vi "LIA DFD Decimation.vi"(7 "stages":i32, 9 "filter delay":i32, 10 "filter in":T1 {"mSRate_QSettings"."source" items=["Coef a/k"=0, "Coef b/v"=7, "Input"=1, "Output"=2, "Multiplicand"=3, "Product"=4, "Sum"=5, "Delay"=6, "Gain"=8]}, 11 "data in":cdb[](array[numeric])) -> (2 "total decimation":dbl, 3 "decimated data":cdb[](array[numeric]))   [LabVIEW 2017]
uses:
  <vilib>/addons/Digital Filter Design/_Objects.llb/DFD Filter Obj.ctl
  <vilib>/addons/Digital Filter Design/_Objects.llb/DFD Filter Coef.ctl
  <vilib>/addons/Digital Filter Design/_Objects.llb/DFD Filter Structure Type Selector.ctl
  <vilib>/addons/Digital Filter Design/_Objects.llb/dfd_Internal Quantization Settings.ctl
  <vilib>/addons/Digital Filter Design/_Objects.llb/dfd_Internal Quantization Srcs.ctl
  <vilib>/addons/Digital Filter Design/_Objects.llb/DFD Coef Norm Type.ctl
  <vilib>/Analysis/2dsp.llb/Decimate (single shot, CDB).vi
  <vilib>/addons/Digital Filter Design/Process.llb/DFD Filtering (Array).vi
  <vilib>/addons/Digital Filter Design/NI_DigFilterLicensed.lvlib
  <vilib>/Analysis/NI_AALPro.lvlib
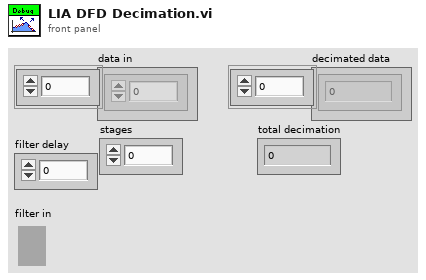
[diagram p1: front panel]
types:
  T1 = typedef "NI_DigFilterLicensed.lvlib/DFD Filter Obj.ctl" = cluster{"mSRate_Fs":dbl, "mSRate_Version":string, "mSRate_Comments":string, "mSRate_OrgCoef":T2, "mSRate_CurCoef":T2, "mSRate_Quantized?":bool, "mSRate_QCoef":T2, "mSRate_QSettings":T4[], "mSRate_Order":i32, "mSRate_Scaling":cluster{"mSRate_ScaleByPowerOf2?":bool, "mSRate_ScaleType":T6}}
  T2 = typedef "NI_DigFilterLicensed.lvlib/DFD Filter Coef.ctl" = cluster{"type":T3, "gain":dbl, "coef a (k)":dbl[], "coef b (v)":dbl[]}
  T3 = typedef "NI_DigFilterLicensed.lvlib/DFD Filter Structure Type Selector.ctl" = enum16{"Undefined", "FIR Direct Form", "FIR Direct Form Transposed", "FIR Symmetric", "FIR Antisymmetric", "IIR Direct Form I", "IIR Direct Form I Transposed", "IIR Direct Form II", "IIR Direct Form II Transposed", "IIR Cascaded Second Order Sections Form I", "IIR Cascaded Second Order Sections Form I Transposed", "IIR Cascaded Second Order Sections Form II", "IIR Cascaded Second Order Sections Form II Transposed", "Lattice Allpass (basic sections)", "Lattice Allpass (one multiplier sections)", "Lattice Allpass (normalized sections)", "Lattice AR (basic sections)", "Lattice AR (one multiplier sections)", "Lattice AR (normalized sections)", "Lattice MA (minimum phase)", "Lattice MA (maximum phase)", "Lattice ARMA (basic sections)", "Lattice ARMA (one multiplier sections)", "Lattice ARMA (normalized sections)"}
  T4 = typedef "NI_DigFilterLicensed.lvlib/dfd_Internal Quantization Settings.ctl" = cluster{"source":T5, "wl":i16, "iwl":i16, "overflow mode":enum16{"Saturation", "Wrap"}, "rounding mode":enum16{"Nearest", "Truncation"}, "signed?":bool}
  T5 = typedef "NI_DigFilterLicensed.lvlib/dfd_Internal Quantization Srcs.ctl" = u16
  T6 = typedef "NI_DigFilterLicensed.lvlib/DFD Coef Norm Type.ctl" = enum16{"No Norm", "Time Domain 1-Norm", "Time Domain 2-Norm", "Time Domain Inf-Norm"}
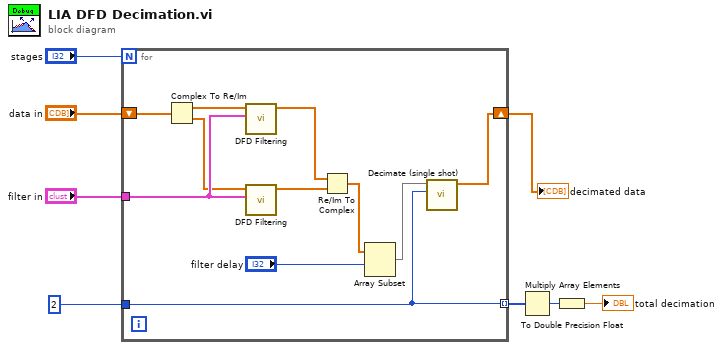
[diagram p0: block diagram]
diagram:
  n1 = for {
    N: "stages" -> [_]
    tunnel: "filter in" -> [w18]
    tunnel: 2 ("value") -> [w12]
    shift-right: [w9] -> w8
    shift-left: "data in" -> [w19]
    tunnel: [w12] -> w4 mode=indexing
    n2 = Complex To Re/Im(x + iy=w19) -> (x=w13:dbl[], y=w14:dbl[])
    n3 = call-poly <vilib>:"DFD Filtering.vi"("filter"=w18, "signal in"=w13) -> ("signal out"=w15:dbl[])  [unwired: 8 in, 1 out]
    n4 = call-poly <vilib>:"DFD Filtering.vi"("filter"=w18, "signal in"=w14) -> ("signal out"=w16:dbl[])  [unwired: 8 in, 1 out]
    n5 = Re/Im To Complex(1:w16, 2:w15) -> (0:w11:cdb[])
    n6 = Array Subset(array=w11, index="filter delay") -> (w10:cdb[])  [unwired: 1 in]
    n7 = call-poly <vilib>:"Decimate (single shot).vi"("decimating factor"=w12, "X"=w10) -> ("Decimated Array"=w9:cdb[])  [unwired: 8 in, 1 out]
  }
  "decimated data" <- w8
  n8 = Multiply Array Elements(1:w4) -> (0:w3:i32)
  n9 = To Double Precision Float(number=w3) -> (double precision float=→"total decimation":dbl)
